vi "Configure AC Current.vi"(0 "VISA resource name":refnum<visa-resource-name>, 1 "NPLC":u16(ring)=1 items=["0.00005", "1", "12", "15"], 5 "Auto Range? (T: Auto)":bool, 7 "Manual Range":dbl=3.0, 9 "Aperture Seconds":dbl, 11 "error in (no error)":errorcluster, 12 "Bandwidth (30)":u16(ring) items=["3", "30", "300"]) -> (4 "VISA resource name out":refnum<visa-resource-name>, 15 "error out":errorcluster)   [LabVIEW 2016, in "Keithley DMM7510.lvlib"]
doc: "This VI configures the AC Current measurement and the related parameters."
uses:
  Keithley DMM7510.lvlib
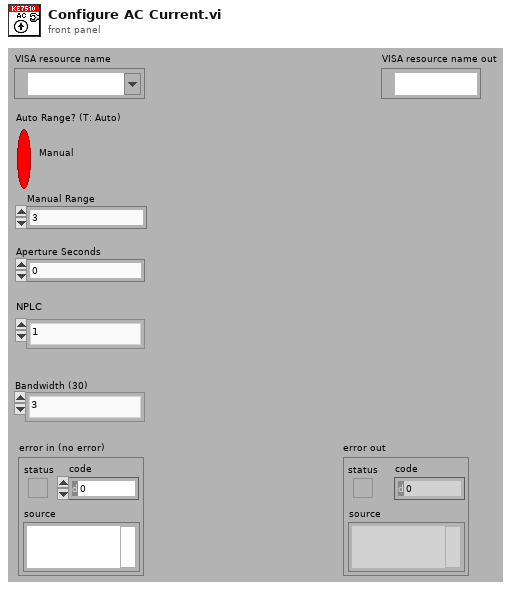
[diagram p1: front panel]
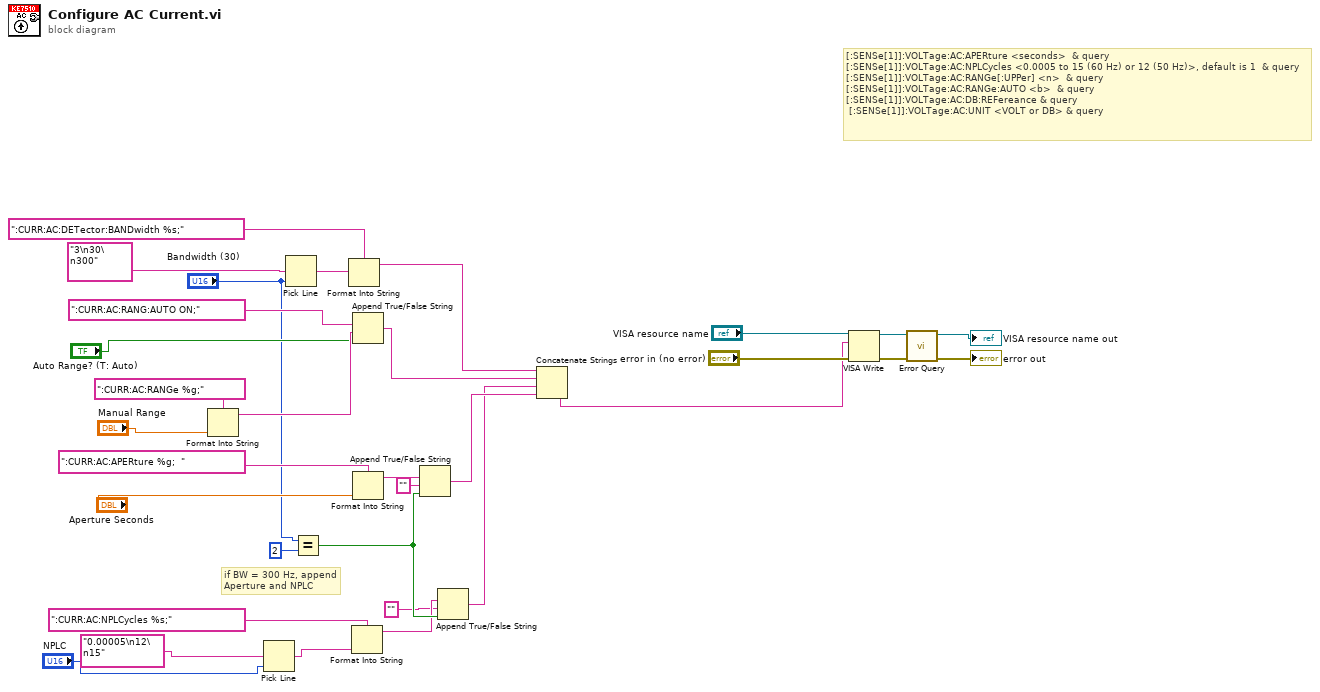
[diagram p0: block diagram]
diagram:
  # "if BW = 300 Hz, append\nAperture and NPLC"
  # "[:SENSe[1]]:VOLTage:AC:APERture <seconds>  & query\n[:SENSe[1]]:VOLTage:AC:NPLCycles <0.0005 to 15 (60 Hz) or 12 (50 Hz)>, default is 1  & query\n[:SENSe[1]]:VOLTage:AC:RANGe[:UPPer] <n>  & query\n[:SENSe[1]]:VOLTage:AC:RANGe:AUTO <b>  & query\n[:SENSe[1]]:VOLTage:AC:DB:REFereance & query\n [:SENSe[1]]:VOLTage:AC:UNIT <VOLT or DB> & query"
  n1 = Format Into String(format string=":CURR:AC:RANGe %g;", "Manual Range") -> (resulting string=w27:string)  [unwired: 2 in, 1 out]
  n2 = Pick Line(multi-line string="0.00005\n12\n15", line index="NPLC") -> (output string=w14:string)  [unwired: 1 in]
  n3 = Pick Line(multi-line string="3\n30\n300", line index="Bandwidth (30)") -> (output string=w17:string)  [unwired: 1 in]
  n4 = Equal?(x="Bandwidth (30)", y=u16 2) -> (x = y?=w4:bool)
  n5 = Format Into String(format string=":CURR:AC:DETector:BANDwidth %s;", w17) -> (resulting string=w24:string)  [unwired: 2 in, 1 out]
  n6 = Format Into String(format string=":CURR:AC:NPLCycles %s;", w14) -> (resulting string=w2:string)  [unwired: 2 in, 1 out]
  n7 = Append True/False String(1:"Auto Range? (T: Auto)", 2:w27, 3:":CURR:AC:RANG:AUTO ON;") -> (0:w23:string)  [unwired: 1 in]
  n8 = Format Into String(format string=":CURR:AC:APERture %g;  ", "Aperture Seconds") -> (resulting string=w7:string)  [unwired: 2 in, 1 out]
  n9 = Append True/False String(1:w4, 2:"" ("false string"), 3:w7) -> (0:w8:string)  [unwired: 1 in]
  n10 = Append True/False String(1:w4, 2:"" ("false string"), 3:w2) -> (0:w3:string)  [unwired: 1 in]
  n11 = Concatenate Strings(w24, w23, w3, w8) -> (w22:string)
  n12 = VISA Write(VISA resource name="VISA resource name", write buffer=w22, error in (no error)="error in (no error)") -> (VISA resource name out=w21:refnum<visa-resource-name>, error out=w20:errorcluster)  [unwired: 1 out]
  n13 = call "Error Query.vi"("error in (no error)"=w20, "VISA resource name"=w21) -> ("error out"=→"error out":errorcluster, "VISA resource name out"=→"VISA resource name out":refnum<visa-resource-name>)  [unwired: 6 in, 2 out]
